vi "Build All.vi"() -> ()   [LabVIEW 2021]
uses:
  <vilib>/AppBuilder/AB_API_Simple/Build (path).vi
  <vilib>/AppBuilder/AB_API_Simple/NI_App_Builder_API.lvlib
panel:
  in  "Linux x64":bool=TRUE
  in  "Linux ARM":bool=TRUE
  in  "Pharlap":bool=TRUE
  in  "Windows":bool=TRUE
  in  "System Configuration":bool=TRUE
  out "String":string
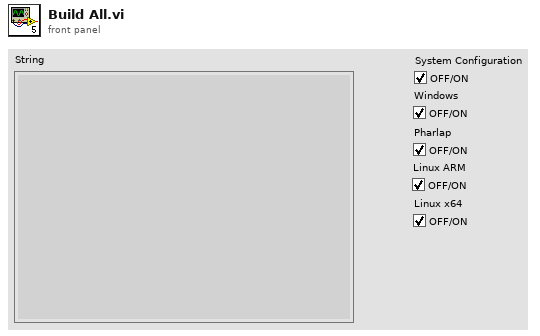
[diagram p1: front panel]
types:
  T1 = cluster{"Display Name":string, "Build Spec Name":string, "Project Name":string, "Target Name":string}[]
  T2 = cluster{"Display Name":string, "Build Spec Name":string, "Project Name":string, "Target Name":string}
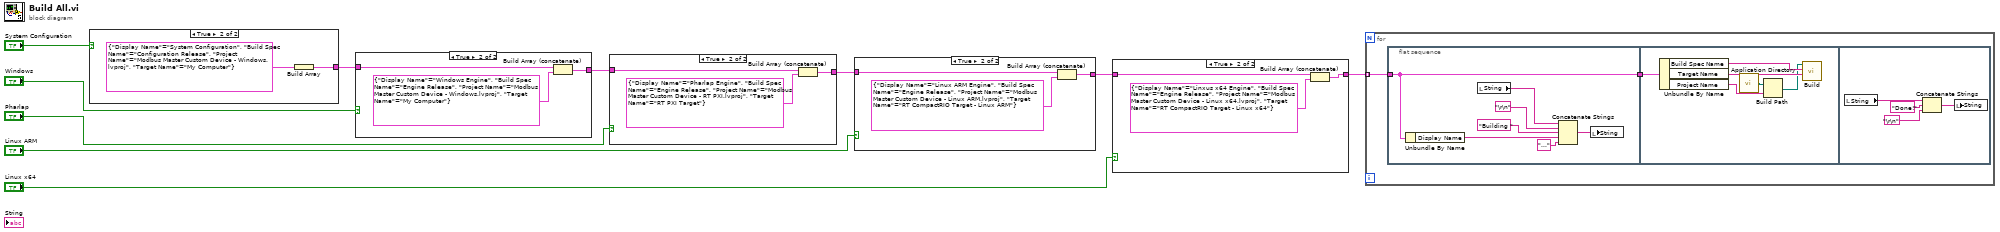
[diagram p0: block diagram]
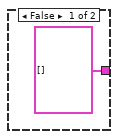
[diagram p6: hidden frame]
diagram:
  n1 = case shown="True" "System Configuration" {
    tunnel: [T1 [] w12] -> w8
    frame False {
    }
    frame True {
      n2 = Build Array(T2 {"Display Name"="System Configuration", "Build Spec Name"="Configuration Release", "Project Name"="Modbus Master Custom Device - Windows.lvproj", "Target Name"="My Computer"} ("Cluster")) -> (w12:T1)
    }
  }
  n3 = case shown="True" "Windows" {
    tunnel: w8 -> [w14 w16]
    tunnel: [w14 w15] -> w6
    frame False {
    }
    frame True {
      n4 = Build Array (concatenate)(w16, T2 {"Display Name"="Windows Engine", "Build Spec Name"="Engine Release", "Project Name"="Modbus Master Custom Device - Windows.lvproj", "Target Name"="My Computer"} ("Cluster")) -> (w15:T1)
    }
  }
  n5 = case shown="True" "Pharlap" {
    tunnel: w6 -> [w18 w20]
    tunnel: [w18 w19] -> w5
    frame False {
    }
    frame True {
      n6 = Build Array (concatenate)(w20, T2 {"Display Name"="Pharlap Engine", "Build Spec Name"="Engine Release", "Project Name"="Modbus Master Custom Device - RT PXI.lvproj", "Target Name"="RT PXI Target"} ("Cluster")) -> (w19:T1)
    }
  }
  n7 = case shown="True" "Linux ARM" {
    tunnel: w5 -> [w22 w24]
    tunnel: [w22 w23] -> w4
    frame False {
    }
    frame True {
      n8 = Build Array (concatenate)(w24, T2 {"Display Name"="Linux ARM Engine", "Build Spec Name"="Engine Release", "Project Name"="Modbus Master Custom Device - Linux ARM.lvproj", "Target Name"="RT CompactRIO Target - Linux ARM"} ("Cluster")) -> (w23:T1)
    }
  }
  n9 = case shown="True" "Linux x64" {
    tunnel: w4 -> [w26 w29]
    tunnel: [w26 w27] -> w3
    frame False {
    }
    frame True {
      n10 = Build Array (concatenate)(w29, T2 {"Display Name"="Linxus x64 Engine", "Build Spec Name"="Engine Release", "Project Name"="Modbus Master Custom Device - Linux x64.lvproj", "Target Name"="RT CompactRIO Target - Linux x64"} ("Cluster")) -> (w27:T1)
    }
  }
  n11 = for {
    tunnel: w3 -> [w31] mode=indexing
    n12 = flat-sequence {
      tunnel: w31 -> [w33]
      tunnel: [w33] -> w30
      tunnel: w30 -> [w44]
      frame #0 {
        n13 = Unbundle By Name(w33) -> ("Display Name"=w36:string)
        n14 = local read "String"() -> (w32:string)
        n15 = Concatenate Strings(w32, "\r\n", "Building " ("string"), w36, "..." ("string")) -> (w34:string)
        n16 = local write "String"(w34) -> ()
      }
      frame #1 {
        n17 = Unbundle By Name(w44) -> ("Build Spec Name"=w43:string, "Target Name"=w42:string, "Project Name"=w40:string)
        n18 = call <vilib>:"Application Directory.vi"() -> ("Application Directory"=w41:path)
        n19 = Build Path(base path=w41, name or relative path=w40) -> (appended path=w39:path)
        n20 = call-poly <vilib>:"Build.vi"("Name of target (My Computer)"=w42, "Name of build specification (if empty: build all)"=w43, "Path to project"=w39) -> ()  [unwired: 7 in, 2 out]
      }
      frame #2 {
        n21 = local read "String"() -> (w45:string)
        n22 = Concatenate Strings(w45, "Done!" ("String"), "\r\n") -> (w47:string)
        n23 = local write "String"(w47) -> ()
      }
    }
  }
